vi "New Digital Reader Actor.vi"(8 "error in (no error)":errorcluster, 9 "Loop Period in ms (20)":u32=20, 10 "DAQmx Task":refnum<k21>, 11 "Digital Reader in":refnum<class "Digital Reader.lvclass">) -> (0 "error out":errorcluster, 3 "Digital Reader out":refnum<class "Digital Reader.lvclass">)   [LabVIEW 2024, in "DAQmx Actor.lvlib" / "Digital Reader.lvclass"]
uses:
  Digital Reader.lvclass
  Digital Reader.lvclass/Digital Reader.ctl
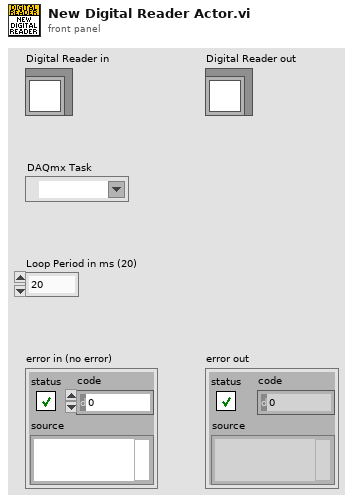
[diagram p1: front panel]
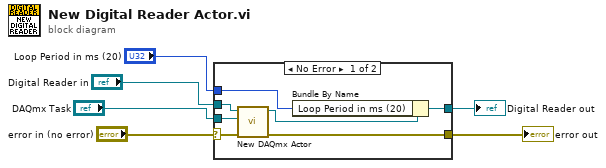
[diagram p0: block diagram]
diagram:
  n1 = case shown="No Error" "error in (no error)" {
    selector: "error in (no error)" -> [w9 w15]
    tunnel: [w8 w15] -> w5
    tunnel: [w7 w14] -> w3
    tunnel: "Digital Reader in" -> [w13 w14]
    tunnel: "DAQmx Task" -> [w12 _]
    tunnel: "Loop Period in ms (20)" -> [w10 _]
    frame No Error {
      n2 = call-dynamic "New DAQmx Actor.vi"("error in (no error)"=w9, "DAQmx Task"=w12, "DAQmx Actor in"=w13) -> ("error out"=w8:errorcluster, "DAQmx Actor out"=w11:refnum<class "Digital Reader.lvclass">)  [unwired: 7 in]
      n3 = Bundle By Name(cluster=w11, "Loop Period in ms (20)"=w10) -> (w7:refnum<class "Digital Reader.lvclass">)
    }
    frame Error {
    }
  }
  "error out" <- w5
  "Digital Reader out" <- w3
